vi "CPP_FFTBoost.vi"(5 "CutoffFrequency":dbl=200.0, 7 "MaxBoost":dbl=15.0, 8 "dF":dbl, 9 "UnwrappedPhaseLag":dbl[](array[numeric]), 10 "AmplitudeBoost":dbl[](array[numeric]), 11 "Muffleddata":dbl[](array[numeric])) -> (1 "BandLimitedBoost":dbl[](array[numeric]), 3 "boostedData":dbl[](array[numeric]), 4 "CutoffFrequencyUsed":dbl=15.0, 6 "MaxBoostUsed":dbl=15.0)   [LabVIEW 2011]
uses:
  <vilib>/Analysis/2dsp.llb/Real FFT.vi
  <vilib>/Analysis/2dsp.llb/Inverse Real FFT.vi
  <vilib>/Analysis/NI_AALPro.lvlib
panel:
  in  "PhaseCorrection":bool=TRUE
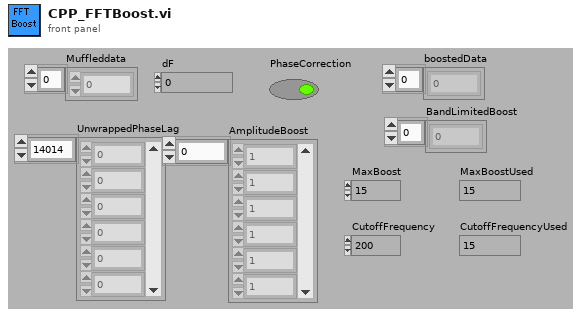
[diagram p1: front panel]
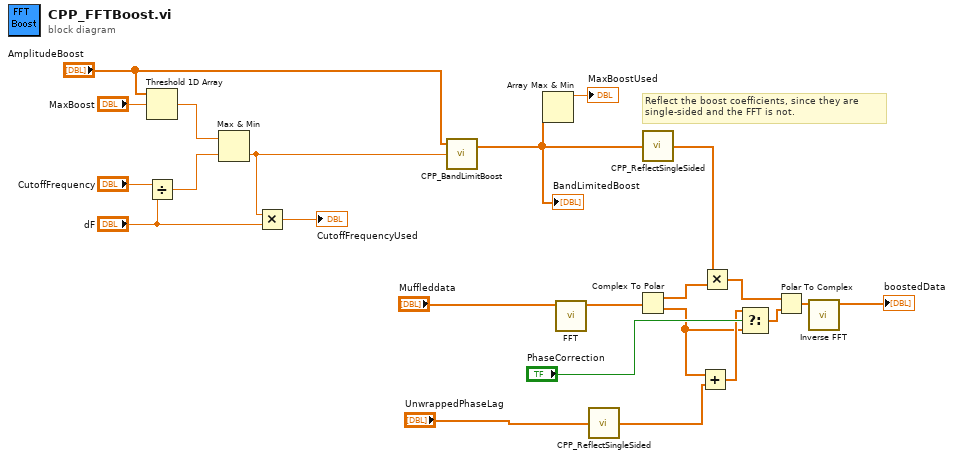
[diagram p0: block diagram]
diagram:
  # "Reflect the boost coefficients, since they are single-sided and the FFT is not."
  n1 = Threshold 1D Array(2:"MaxBoost", 3:"AmplitudeBoost") -> (0:w13:dbl)  [unwired: 1 in]
  n2 = Divide(x="CutoffFrequency", y="dF") -> (x/y=w14:dbl)
  n3 = Max & Min(x=w13, y=w14) -> (min(x,y)=w10:dbl)  [unwired: 1 out]
  n4 = Multiply(x=w10, y="dF") -> (x*y=→"CutoffFrequencyUsed":dbl)
  n5 = call "CPP_BandLimitBoost.vi"("CutoffIndex"=w10, "AmplitudeBoost"="AmplitudeBoost") -> ("BandLimitedBoost"=w6:dbl[])  [unwired: 2 in]
  "BandLimitedBoost" <- w6
  n6 = Array Max & Min(array=w6) -> (max value=→"MaxBoostUsed":dbl)  [unwired: 3 out]
  n7 = call-poly <vilib>:"FFT.vi"("X"="Muffleddata") -> ("FFT {X}"=w19:cdb[])  [unwired: 9 in, 1 out]
  n8 = call "CPP_ReflectSingleSided.vi"("SingleSidedData"="UnwrappedPhaseLag") -> ("ReflectedData"=w17:dbl[])
  n9 = Complex To Polar(r * e^(i*theta)=w19) -> (r=w20:dbl[], theta=w1:dbl[])
  n10 = call "CPP_ReflectSingleSided.vi"("SingleSidedData"=w6) -> ("ReflectedData"=w9:dbl[])
  n11 = Add(x=w1, y=w17) -> (x+y=w3:dbl[])
  n12 = Multiply(x=w9, y=w20) -> (x*y=w21:dbl[])
  n13 = Select(t=w3, s="PhaseCorrection", f=w1) -> (s? t:f=w2:dbl[])
  n14 = Polar To Complex(1:w2, 2:w21) -> (0:w22:cdb[])
  n15 = call-poly <vilib>:"Inverse FFT.vi"("FFT {X}"=w22) -> ("X"=→"boostedData":dbl[])  [unwired: 9 in, 1 out]
